vi "ICDAS_LoadPlugin.vi"(8 "error in (no error)":errorcluster, 9 "PathToPluginINI":path, 10 "Module Name":string, 11 "ModuleID":i32) -> (0 "error out":errorcluster)   [LabVIEW 2018]
uses:
  <vilib>/Utility/error.llb/Error Cluster From Error Code.vi
  <vilib>/ErrorRing/Error Ring.xnode
  NistPluggableModules/Sync/SyncPlugins/SyncPluginBase/SyncPluginBase.lvclass
  NistPluggableModules/FGen/FgenPlugins/FgenPluginBaseClass/FgenPluginsBase.lvclass
  NistPluggableModules/Scope/ScopeModule/ScopeModule.lvlib
  NistPluggableModules/Digitizer/DigitizerPlugins/DigitizerBaseClass/DigitizerBase.lvclass
  NistPluggableModules/Sensor/SensorModule/SensorModule.lvlib
  NistPluggableModules/Analysis/AnalysisPlugins/AnalysisPluginBaseClass/AnalysisPluginsBase.lvclass
  NistPluggableModules/AcPwr/AcPwrModule/AcPwrModule.lvlib
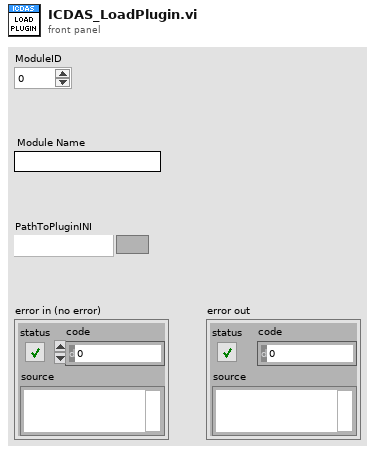
[diagram p1: front panel]
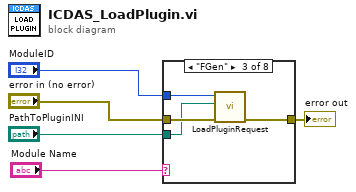
[diagram p0: block diagram]
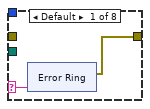
[diagram p2: hidden frame]
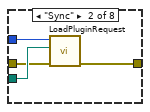
[diagram p3: hidden frame]
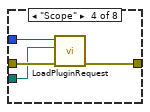
[diagram p4: hidden frame]
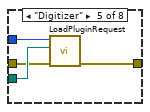
[diagram p5: hidden frame]
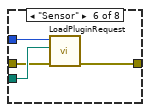
[diagram p6: hidden frame]
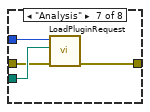
[diagram p7: hidden frame]
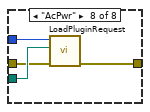
[diagram p8: hidden frame]
diagram:
  n1 = case shown="\"FGen\"" "Module Name" {
    selector: "Module Name" -> [w7 _ _ _ _ _ _ _]
    tunnel: "ModuleID" -> [_ w18 w19 w23 w30 w34 w38 w42]
    tunnel: "PathToPluginINI" -> [_ w17 w20 w24 w29 w33 w37 w41]
    tunnel: "error in (no error)" -> [_ w16 w22 w25 w28 w32 w36 w40]
    tunnel: [w6 w15 w21 w26 w27 w31 w35 w39] -> w5
    frame Default {
      n2 = xnode "Error Ring"("parameter 0"=w7) -> ("error out"=w6:errorcluster)
    }
    frame "Sync" {
      n3 = call "LoadPluginRequest.vi"("error in (no error)"=w16, "PathToPluginINI"=w17, "ModuleID"=w18) -> ("error out"=w15:errorcluster)  [unwired: 8 in]
    }
    frame "FGen" {
      n4 = call "LoadPluginRequest.vi"("error in (no error)"=w22, "PathToPluginINI"=w20, "ModuleID"=w19) -> ("error out"=w21:errorcluster)  [unwired: 8 in]
    }
    frame "Scope" {
      n5 = call "LoadPluginRequest.vi"("error in (no error)"=w25, "PathToPluginINI"=w24, "ModuleID"=w23) -> ("error out"=w26:errorcluster)  [unwired: 8 in]
    }
    frame "Digitizer" {
      n6 = call "LoadPluginRequest.vi"("error in (no error)"=w28, "PathToPluginINI"=w29, "ModuleID"=w30) -> ("error out"=w27:errorcluster)  [unwired: 8 in]
    }
    frame "Sensor" {
      n7 = call "LoadPluginRequest.vi"("error in (no error)"=w32, "PathToPluginINI"=w33, "ModuleID"=w34) -> ("error out"=w31:errorcluster)  [unwired: 8 in]
    }
    frame "Analysis" {
      n8 = call "LoadPluginRequest.vi"("error in (no error)"=w36, "PathToPluginINI"=w37, "ModuleID"=w38) -> ("error out"=w35:errorcluster)  [unwired: 8 in]
    }
    frame "AcPwr" {
      n9 = call "LoadPluginRequest.vi"("error in (no error)"=w40, "PathToPluginINI"=w41, "ModuleID"=w42) -> ("error out"=w39:errorcluster)  [unwired: 8 in]
    }
  }
  "error out" <- w5
